vi "lijnvolgen manueel afstandssensor.vi"() -> ()   [LabVIEW 2019]
uses:
  <vilib>/myRIO/Common/Instrument Driver Framework/Utilities/typedefs/Analog Scaling Constants.ctl
  <vilib>/myRIO/Common/Instrument Driver Framework/Utilities/typedefs/Analog Scaling Constants List.ctl
  <vilib>/myRIO/Common/Instrument Driver Framework/myRIO v1.0/AO/typedefs/AO Channels Enum.ctl
  <vilib>/myRIO/Common/Instrument Driver Framework/myRIO v1.0/AO/typedefs/AO Channels List.ctl
  <vilib>/myRIO/Common/Instrument Driver Framework/Utilities/typedefs/Generic FPGA Reference.ctl
  <vilib>/myRIO/Common/Instrument Driver Framework/Utilities/typedefs/myRIO v1.0 Reference.ctl
  <vilib>/myRIO/Common/Instrument Driver Framework/Utilities/typedefs/Hardware Version Enum.ctl
  <vilib>/myRIO/Common/Instrument Driver Framework/Utilities/typedefs/myRIO Generic Hardware Reference.ctl
  <vilib>/myRIO/Instrument Drivers/Onboard IO/AO/typedefs/AO Reference.ctl
  <vilib>/myRIO/Instrument Drivers/Onboard IO/AO/AO.lvlib
  <vilib>/myRIO/Instrument Drivers/Onboard IO/AO/vis/Write.vi
  <vilib>/userDefined/High Color/nirio_resource_hc.ctl
  <vilib>/myRIO/Common/Instrument Driver Framework/myRIO v1.0/AO/vis/myRIO v1.1 Open AO.vi
  <vilib>/myRIO/Instrument Drivers/Onboard IO/AO/vis/myRIO AO Open.xnode
  <vilib>/myRIO/Common/Instrument Driver Framework/Utilities/vis/Is FPGA Ref Available.vi
  <vilib>/myRIO/Express VI/Onboard IO/AO/AO Express VI.xnode
  <vilib>/myRIO/Common/Instrument Driver Framework/myRIO v1.0/AI/typedefs/AI Channels Enum.ctl
  <vilib>/myRIO/Common/Instrument Driver Framework/myRIO v1.0/AI/typedefs/AI Channels List.ctl
  <vilib>/myRIO/Instrument Drivers/Onboard IO/AI/typedefs/AI Reference.ctl
  <vilib>/myRIO/Instrument Drivers/Onboard IO/AI/AI.lvlib
  <vilib>/myRIO/Instrument Drivers/Onboard IO/AI/vis/Read.vi
  <vilib>/myRIO/Common/Instrument Driver Framework/myRIO v1.0/AI/vis/myRIO v1.1 Open AI.vi
  <vilib>/myRIO/Instrument Drivers/Onboard IO/AI/vis/myRIO AI Open.xnode
  <vilib>/myRIO/Express VI/Onboard IO/AI/AI Express VI.xnode
  <vilib>/myRIO/Common/Instrument Driver Framework/myRIO v1.0/DIO/typedefs/DIO Channels Enum.ctl
  <vilib>/myRIO/Common/Instrument Driver Framework/myRIO v1.0/DIO/typedefs/DIO Channels List.ctl
  <vilib>/myRIO/Instrument Drivers/Onboard IO/DIO/typedefs/DIO Reference.ctl
  <vilib>/myRIO/Instrument Drivers/Onboard IO/DIO/DIO.lvlib
  <vilib>/myRIO/Instrument Drivers/Onboard IO/DIO/vis/Read.vi
  <vilib>/myRIO/Common/Instrument Driver Framework/myRIO v1.0/DIO/vis/myRIO v1.1 Open DIO.vi
  <vilib>/myRIO/Instrument Drivers/Onboard IO/DIO/vis/myRIO DIO Open.xnode
  <vilib>/myRIO/Express VI/Onboard IO/DI/DI Express VI.xnode
  Globalmanueel.vi
  <vilib>/myRIO/Instrument Drivers/Onboard IO/DIO/vis/Write.vi
  <vilib>/myRIO/Express VI/Onboard IO/DO/DO Express VI.xnode
panel:
  in  "voorwaarts":bool
  in  "achterwaarts":bool
  in  "links draaien":bool
  in  "rechts draaien":bool
  in  "snelheid":dbl
  in  "links draaien achteruit":bool
  in  "rechts draaien achteruit":bool
  in  "stoppen":bool
  in  "HOOFDWHILELOOP":bool
  out "Numeric 4":i32
  out "analoog":dbl[](array[numeric])
  out "Array 3":i32[](array[numeric])
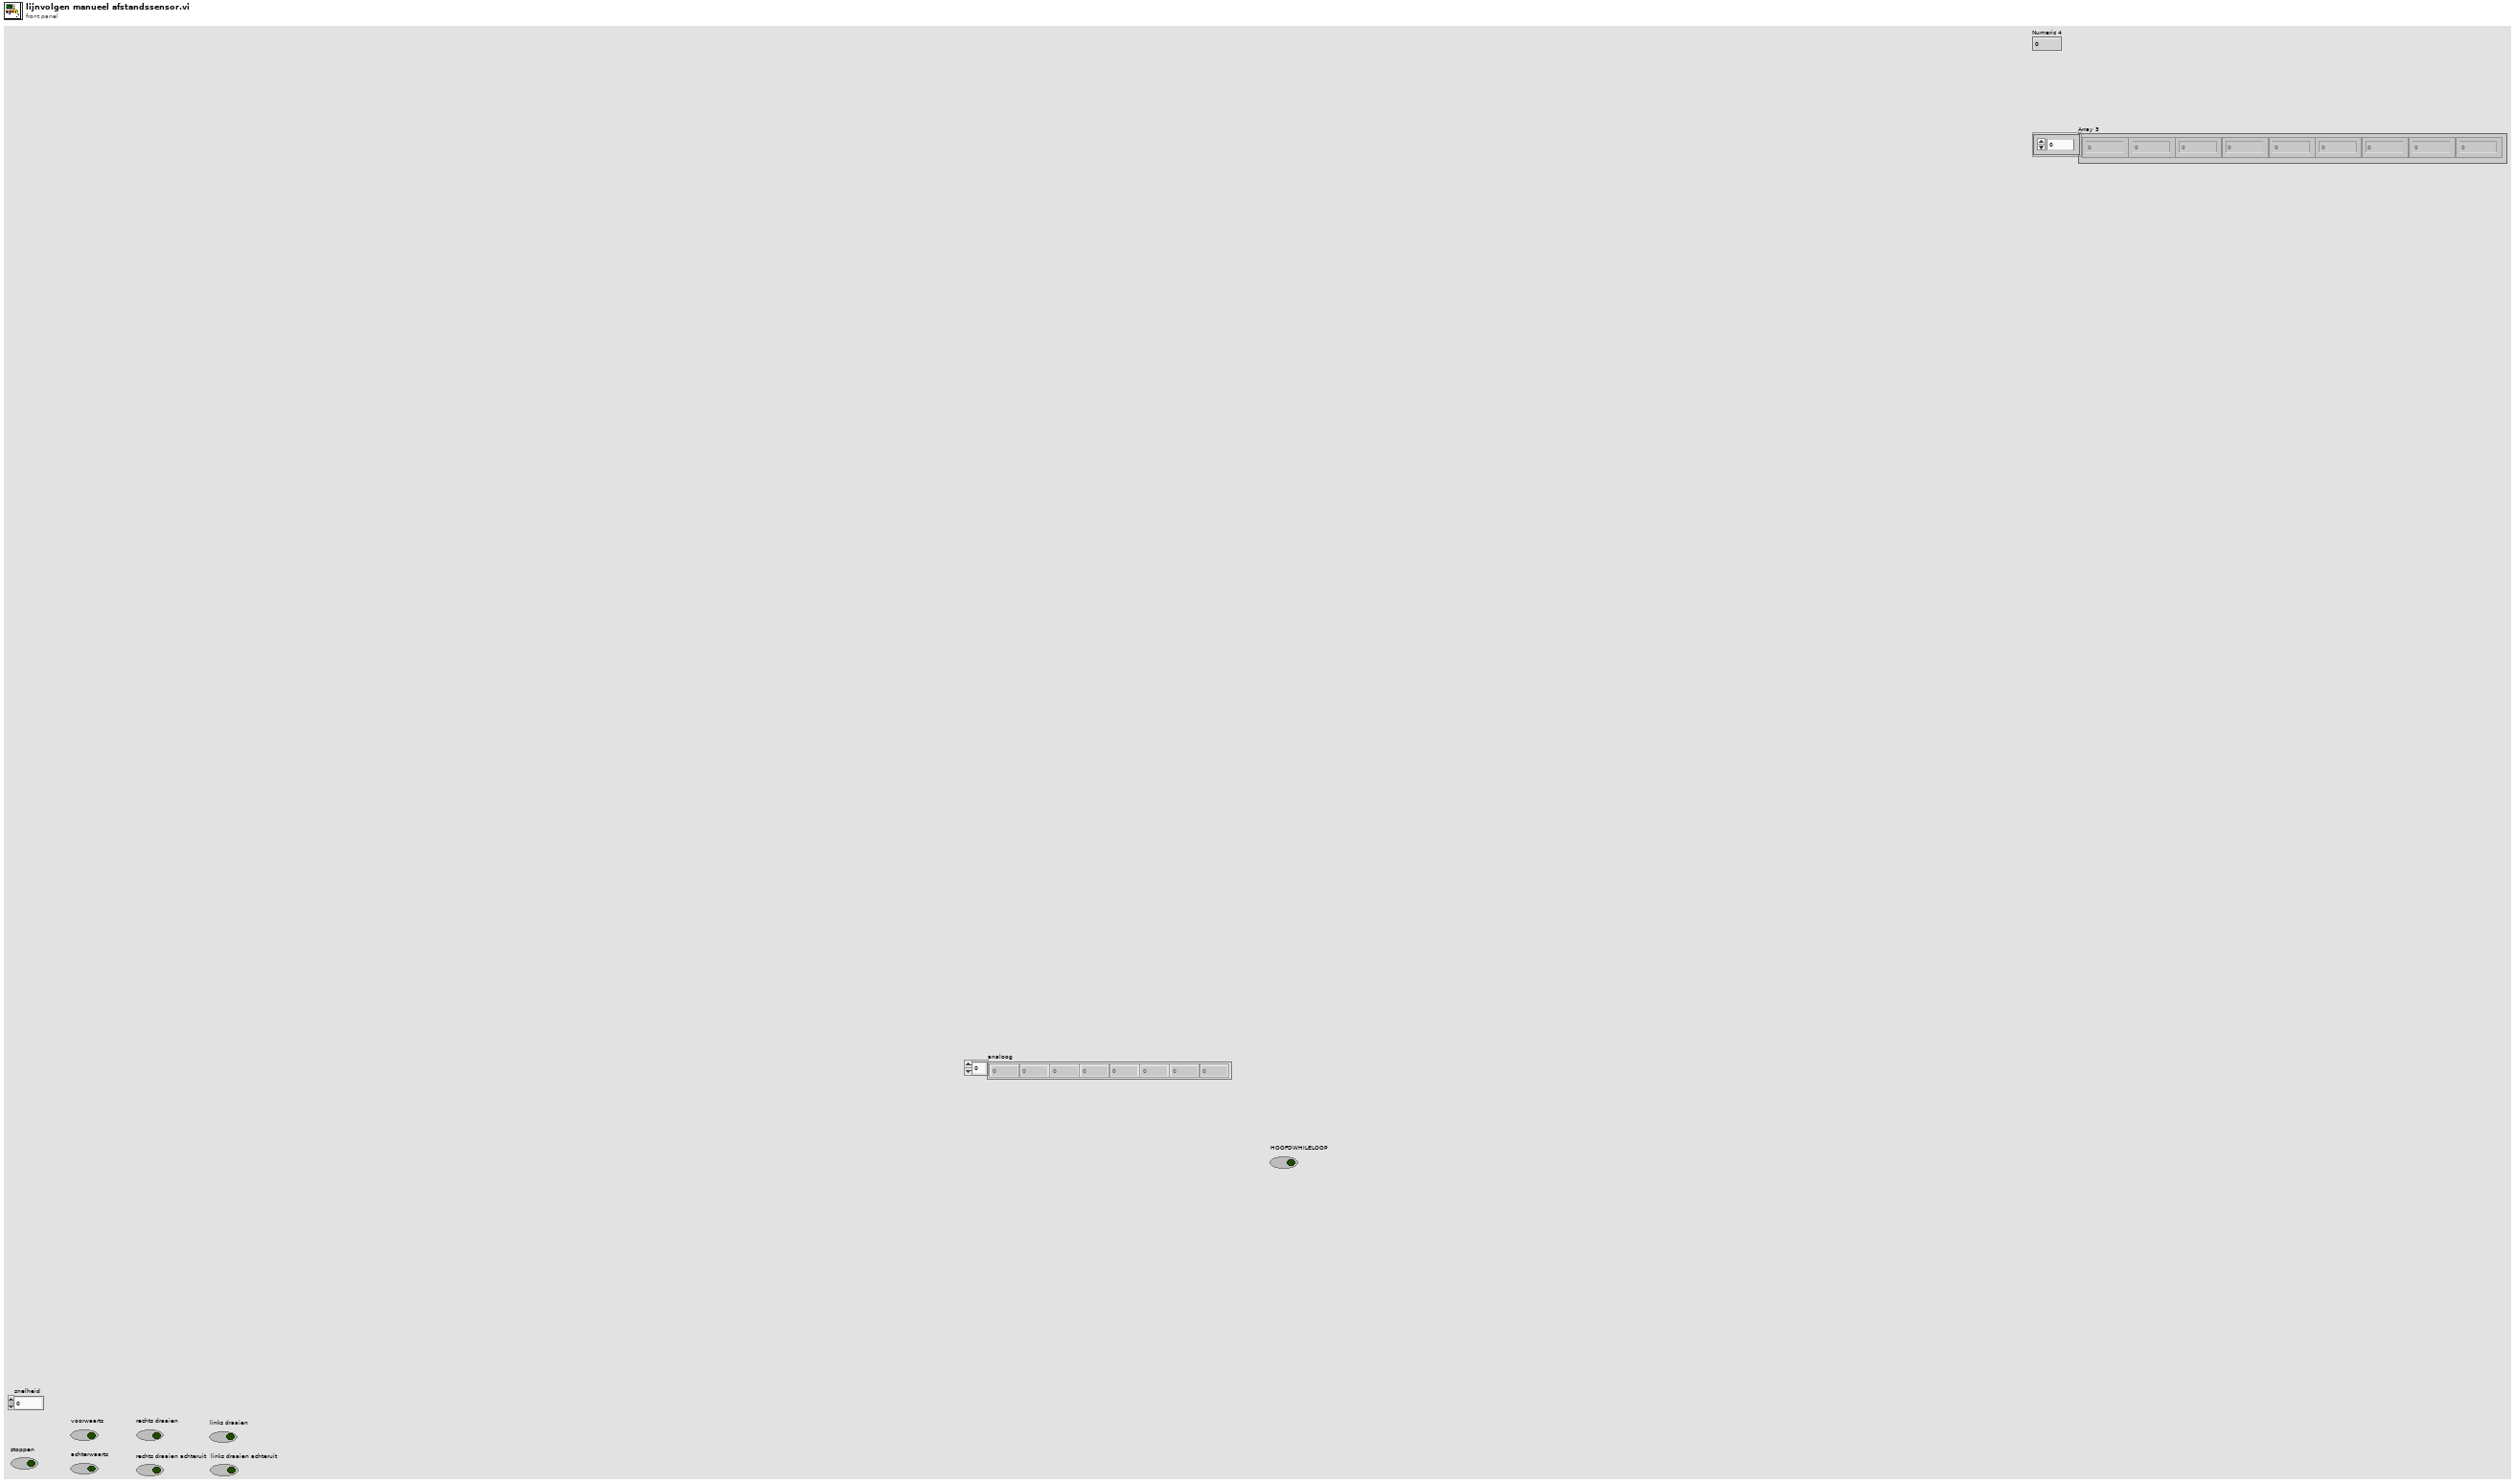
[diagram p1: front panel]
types:
  T1 = typedef "DIO.lvlib/DIO Reference.ctl" = cluster{"myRIO Reference":T2, "DIO Channels List":T6}
  T2 = typedef "myRIO Generic Hardware Reference.ctl" = cluster{"myRIO Model":T3, "myRIO Hardware Reference":T4}
  T3 = typedef "Hardware Version Enum.ctl" = enum16{"Unknown", "myRIO-1900", "myRIO-1950", "roboRIO", "NI ELVIS RIO CM", "ELVIS III"}
  T4 = typedef "myRIO v1.0 Reference.ctl" = cluster{"Generic FPGA Reference":T5, "Allow multiple opens":bool}
  T5 = typedef "Generic FPGA Reference.ctl" = refnum<k20>
  T6 = typedef "DIO Channels List.ctl" = T7[]
  T7 = typedef "DIO Channels Enum.ctl" = enum16{"Not Connected", "C/DIO0", "C/DIO1", "C/DIO2", "C/DIO3", "C/DIO4", "C/DIO5", "C/DIO6", "C/DIO7", "A/DIO0", "A/DIO1", "A/DIO2", "A/DIO3", "A/DIO4", "A/DIO5", "A/DIO6", "A/DIO7", "A/DIO8", "A/DIO9", "A/DIO10", "A/DIO11", "A/DIO12", "A/DIO13", "A/DIO14", "A/DIO15", "A/DIO16", "A/DIO17", "A/DIO18", "A/DIO19", "B/DIO0", "B/DIO1", "B/DIO2", "B/DIO3", "B/DIO4", "B/DIO5", "B/DIO6", "B/DIO7", "B/DIO8", "B/DIO9", "B/DIO10", "B/DIO11", "B/DIO12", "B/DIO13", "B/DIO14", "B/DIO15", "B/DIO16", "B/DIO17", "B/DIO18", "B/DIO19", "LED0", "LED1", "LED2", "LED3", "Button0", "DIO/DIO0", "DIO/DIO1", "DIO/DIO2", "DIO/DIO3", "DIO/DIO4", "DIO/DIO5", "DIO/DIO6", "DIO/DIO7", "DIO/DIO8", "DIO/DIO9", "SPI/CS0", "SPI/CS1", "SPI/CS2", "SPI/CS3", "LED RADIO (Green)", "LED RADIO (Red)", "LED COMM (Green)", "LED COMM (Red)", "LED MODE (Green)", "LED MODE (Red)"}
  T8 = typedef "nirio_resource_hc.ctl" = tag
  T9 = typedef "AO.lvlib/AO Reference.ctl" = cluster{"myRIO Reference":T2, "AO Channel List":T10, "AO Scaling Constant List":T12}
  T10 = typedef "AO Channels List.ctl" = T11[]
  T11 = typedef "AO Channels Enum.ctl" = enum16{"Not Connected", "AudioOut/Left", "AudioOut/Right", "C/AO0", "C/AO1", "A/AO0", "A/AO1", "B/AO0", "B/AO1"}
  T12 = typedef "Analog Scaling Constants List.ctl" = T13[]
  T13 = typedef "Analog Scaling Constants.ctl" = cluster{"LSB Weight (Volts)":dbl, "Offset (Volts)":dbl, "Signed?":bool}
  T14 = typedef "AI.lvlib/AI Reference.ctl" = cluster{"myRIO Reference":T2, "AI Channels List":T15, "AI Scaling Constants List":T12}
  T15 = typedef "AI Channels List.ctl" = T16[]
  T16 = typedef "AI Channels Enum.ctl" = enum16{"Not Connected", "AudioIn/Left", "AudioIn/Right", "C/AI0", "C/AI1", "A/AI0", "A/AI1", "A/AI2", "A/AI3", "A/AI4", "A/AI5", "A/AI6", "A/AI7", "B/AI0", "B/AI1", "B/AI2", "B/AI3", "B/AI4", "B/AI5", "B/AI6", "B/AI7", "AI/AI0", "AI/AI1", "AI/AI2", "AI/AI3", "A/AI0 (DIFF)", "A/AI1 (DIFF)", "A/AI2 (DIFF)", "A/AI3 (DIFF)", "B/AI0 (DIFF)", "B/AI1 (DIFF)", "B/AI2 (DIFF)", "B/AI3 (DIFF)"}
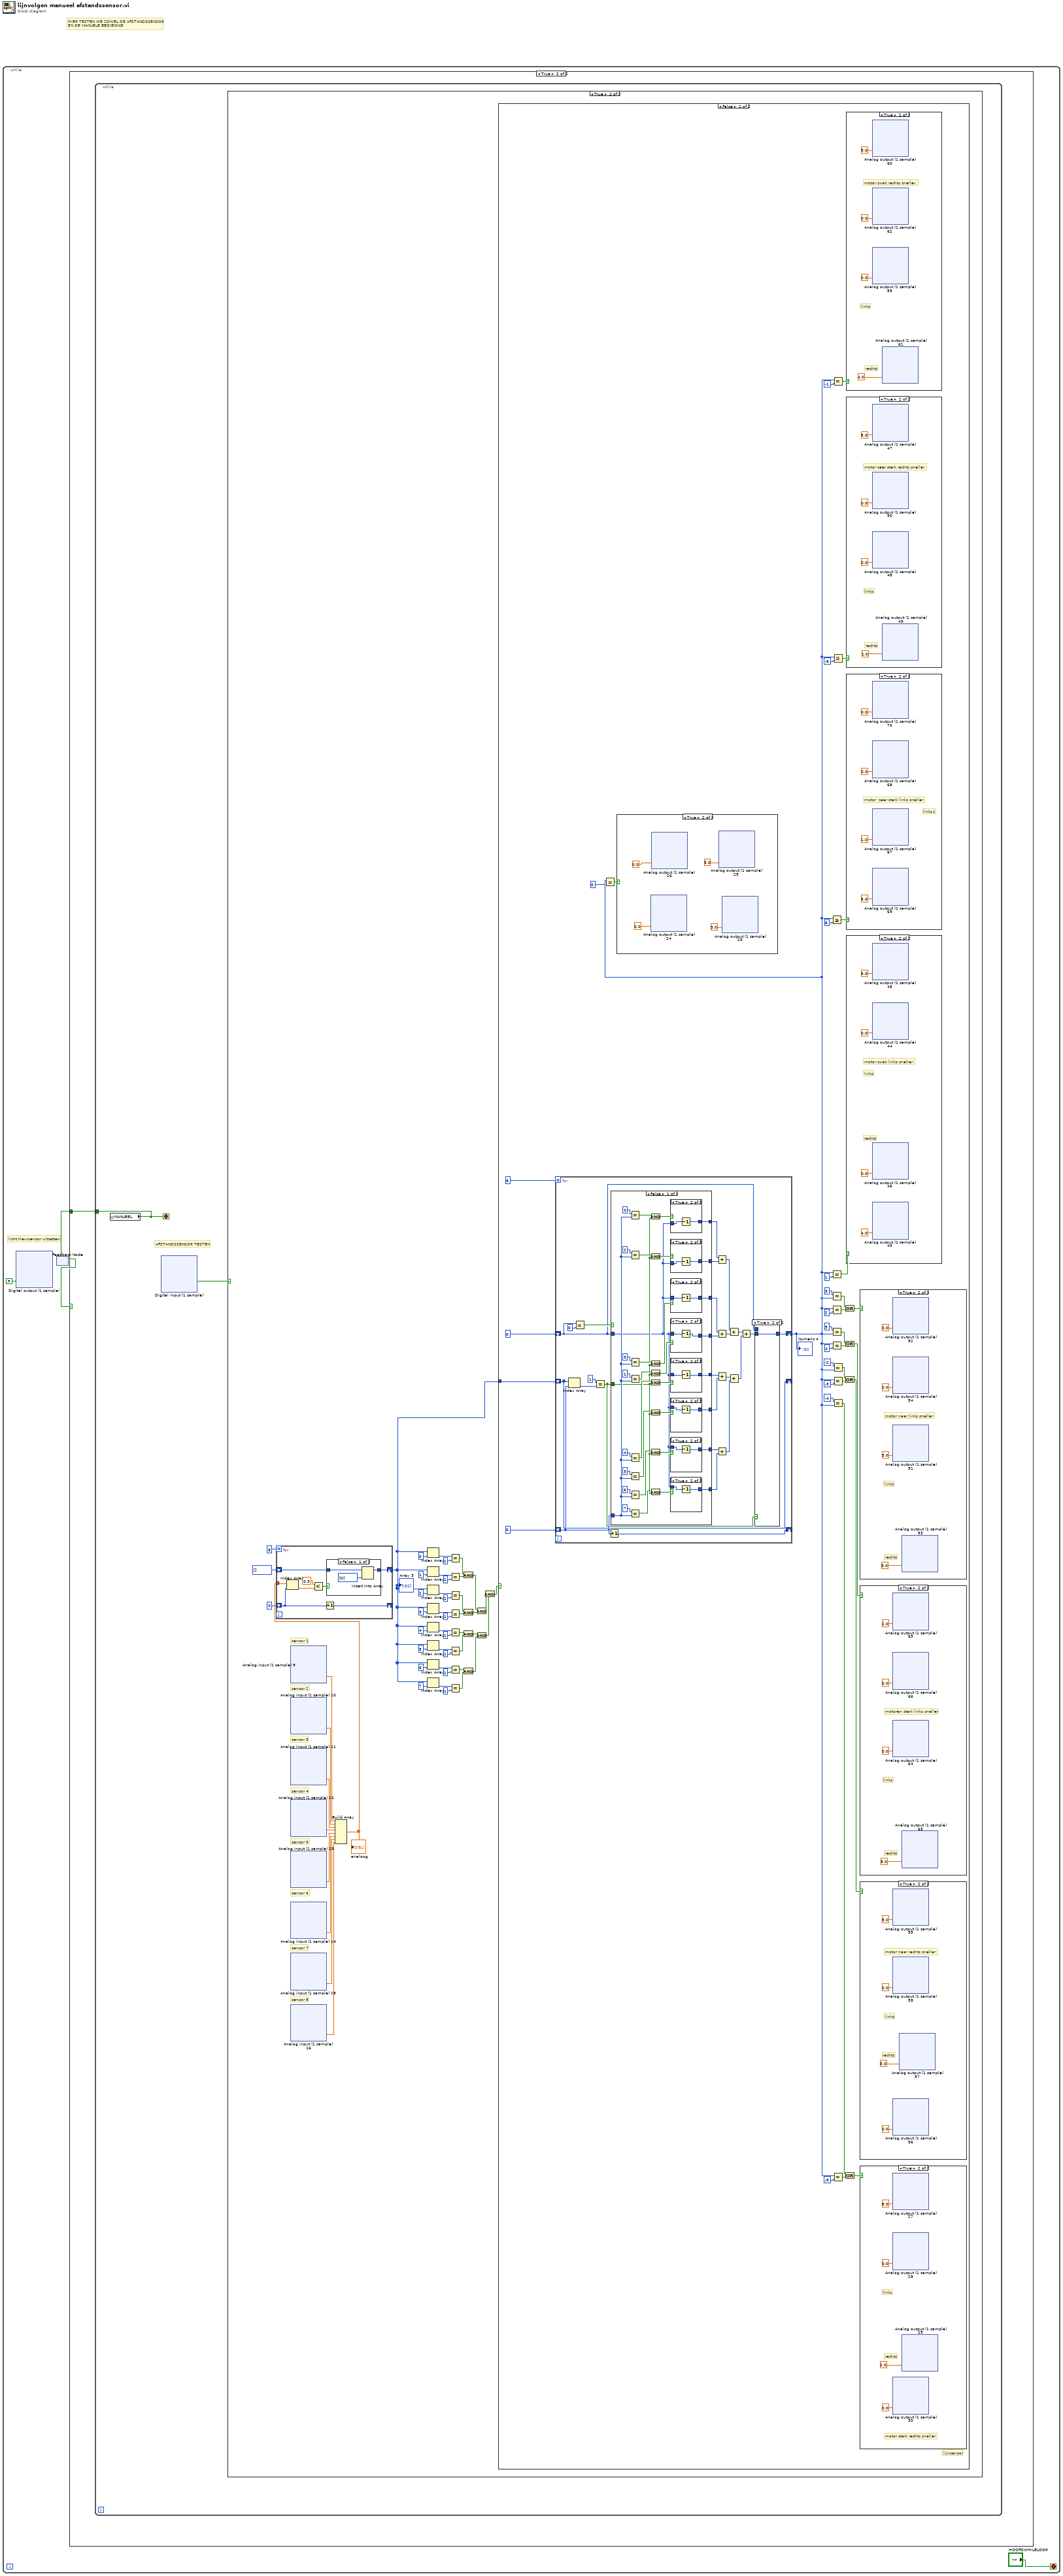
[diagram p0: block diagram]
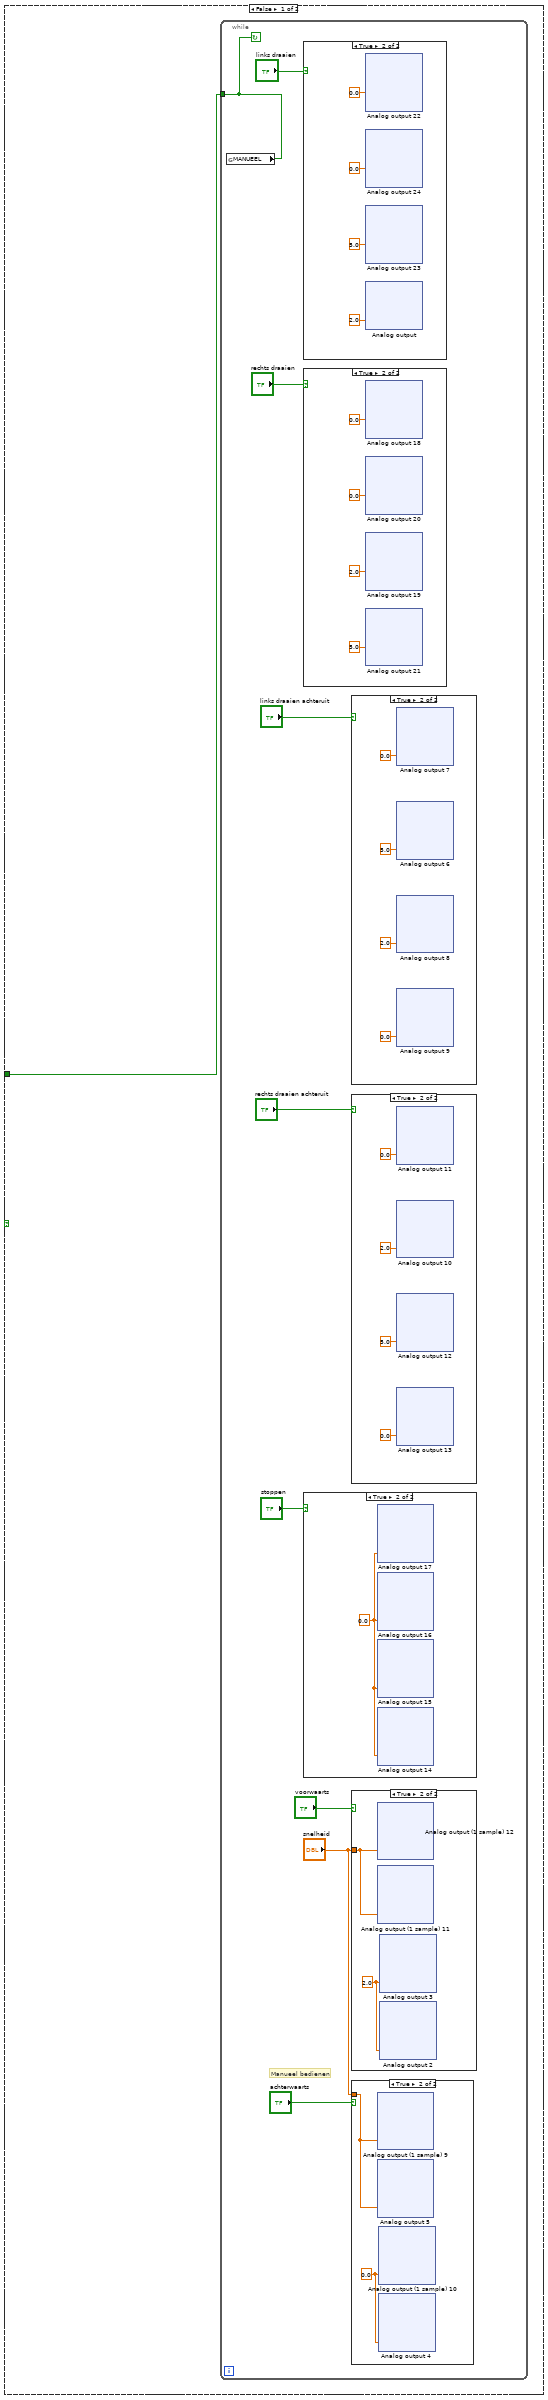
[diagram p2: hidden frame]
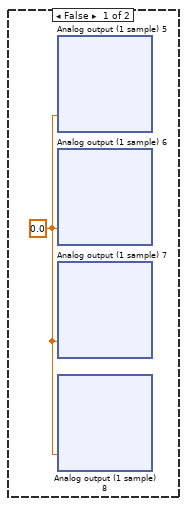
[diagram p10: hidden frame]
diagram:
  # "HIER TESTEN WE ZOWEL DE AFSTANDSSENSOR\nEN DE MANUELE BEDIENING"
  n1 = while {
    stop <- "HOOFDWHILELOOP" stop-if-true
    # "licht kleursensor uitzetten"
    n2 = xnode "Digital output (1 sample)"("A/DIO2 (Pin 15)"=FALSE) -> ()  [unwired: 1 in, 1 out]
    n3 = feedback #1() -> (w1:bool)  [unwired: 1 in]
    n4 = case shown="True" w1 {
      tunnel: [w40 w1107] -> w2
      frame False {
        n5 = while {
          tunnel: [w41] -> w40
          stop <- w41 continue-if-true
          # "Manueel bedienen"
          n6 = global read "Globalmanueel.vi" "MANUEEL"() -> (w41:bool)
          n7 = case shown="True" "links draaien" {
            frame False {
            }
            frame True {
              n8 = xnode "Analog output 22"("B/AO1 (Pin 4)"=0.0) -> ()  [unwired: 1 in, 1 out]
              n9 = xnode "Analog output 24"("A/AO1 (Pin 4)"=0.0) -> ()  [unwired: 1 in, 1 out]
              n10 = xnode "Analog output 23"("B/AO0 (Pin 2)"=5.0) -> ()  [unwired: 1 in, 1 out]
              n11 = xnode "Analog output"("A/AO0 (Pin 2)"=2.0) -> ()  [unwired: 1 in, 1 out]
            }
          }
          n12 = case shown="True" "rechts draaien" {
            frame False {
            }
            frame True {
              n13 = xnode "Analog output 18"("B/AO1 (Pin 4)"=0.0) -> ()  [unwired: 1 in, 1 out]
              n14 = xnode "Analog output 20"("A/AO1 (Pin 4)"=0.0) -> ()  [unwired: 1 in, 1 out]
              n15 = xnode "Analog output 19"("B/AO0 (Pin 2)"=2.0) -> ()  [unwired: 1 in, 1 out]
              n16 = xnode "Analog output 21"("A/AO0 (Pin 2)"=5.0) -> ()  [unwired: 1 in, 1 out]
            }
          }
          n17 = case shown="True" "stoppen" {
            frame False {
            }
            frame True {
              w50 = 0.0
              n18 = xnode "Analog output 17"("A/AO0 (Pin 2)"=w50) -> ()  [unwired: 1 in, 1 out]
              n19 = xnode "Analog output 16"("A/AO1 (Pin 4)"=w50) -> ()  [unwired: 1 in, 1 out]
              n20 = xnode "Analog output 15"("B/AO0 (Pin 2)"=w50) -> ()  [unwired: 1 in, 1 out]
              n21 = xnode "Analog output 14"("B/AO1 (Pin 4)"=w50) -> ()  [unwired: 1 in, 1 out]
            }
          }
          n22 = case shown="True" "links draaien achteruit" {
            frame False {
            }
            frame True {
              n23 = xnode "Analog output 7"("B/AO0 (Pin 2)"=0.0) -> ()  [unwired: 1 in, 1 out]
              n24 = xnode "Analog output 6"("B/AO1 (Pin 4)"=5.0) -> ()  [unwired: 1 in, 1 out]
              n25 = xnode "Analog output 8"("A/AO1 (Pin 4)"=2.0) -> ()  [unwired: 1 in, 1 out]
              n26 = xnode "Analog output 9"("A/AO0 (Pin 2)"=0.0) -> ()  [unwired: 1 in, 1 out]
            }
          }
          n27 = case shown="True" "rechts draaien achteruit" {
            frame False {
            }
            frame True {
              n28 = xnode "Analog output 11"("B/AO0 (Pin 2)"=0.0) -> ()  [unwired: 1 in, 1 out]
              n29 = xnode "Analog output 10"("B/AO1 (Pin 4)"=2.0) -> ()  [unwired: 1 in, 1 out]
              n30 = xnode "Analog output 12"("A/AO1 (Pin 4)"=5.0) -> ()  [unwired: 1 in, 1 out]
              n31 = xnode "Analog output 13"("A/AO0 (Pin 2)"=0.0) -> ()  [unwired: 1 in, 1 out]
            }
          }
          n32 = case shown="True" "voorwaarts" {
            tunnel: "snelheid" -> [_ w957]
            frame False {
            }
            frame True {
              w958 = 2.0
              n33 = xnode "Analog output (1 sample) 12"("A/AO0 (Pin 2)"=w957) -> ()  [unwired: 1 in, 1 out]
              n34 = xnode "Analog output (1 sample) 11"("B/AO0 (Pin 2)"=w957) -> ()  [unwired: 1 in, 1 out]
              n35 = xnode "Analog output 3"("A/AO1 (Pin 4)"=w958) -> ()  [unwired: 1 in, 1 out]
              n36 = xnode "Analog output 2"("B/AO1 (Pin 4)"=w958) -> ()  [unwired: 1 in, 1 out]
            }
          }
          n37 = case shown="True" "achterwaarts" {
            tunnel: "snelheid" -> [_ w807]
            frame False {
            }
            frame True {
              w808 = 0.0
              n38 = xnode "Analog output (1 sample) 9"("A/AO1 (Pin 4)"=w807) -> ()  [unwired: 1 in, 1 out]
              n39 = xnode "Analog output 5"("B/AO1 (Pin 4)"=w807) -> ()  [unwired: 1 in, 1 out]
              n40 = xnode "Analog output (1 sample) 10"("A/AO0 (Pin 2)"=w808) -> ()  [unwired: 1 in, 1 out]
              n41 = xnode "Analog output 4"("B/AO0 (Pin 2)"=w808) -> ()  [unwired: 1 in, 1 out]
            }
          }
        }
      }
      frame True {
        n42 = while {
          tunnel: [w1108] -> w1107
          stop <- w1108 stop-if-true
          # "AFSTANDSSENSOR TESTEN"
          n43 = global read "Globalmanueel.vi" "MANUEEL"() -> (w1108:bool)
          n44 = xnode "Digital input (1 sample)"() -> ("A/DIO1 (Pin 13)"=w1109:bool)  [unwired: 1 in, 1 out]
          n45 = case shown="True" w1109 {
            frame False {
              w1145 = 0.0
              n46 = xnode "Analog output (1 sample) 5"("A/AO0 (Pin 2)"=w1145) -> ()  [unwired: 1 in, 1 out]
              n47 = xnode "Analog output (1 sample) 6"("A/AO1 (Pin 4)"=w1145) -> ()  [unwired: 1 in, 1 out]
              n48 = xnode "Analog output (1 sample) 7"("B/AO0 (Pin 2)"=w1145) -> ()  [unwired: 1 in, 1 out]
              n49 = xnode "Analog output (1 sample) 8"("B/AO1 (Pin 4)"=w1145) -> ()  [unwired: 1 in, 1 out]
            }
            frame True {
              # "sensor 8"
              # "sensor 7"
              # "sensor 6"
              # "sensor 5"
              # "sensor 4"
              # "sensor 3"
              # "sensor 2"
              # "sensor 1"
              n50 = xnode "Analog input (1 sample) 9"() -> ("A/AI3 (Pin 9)"=w1297:dbl)  [unwired: 1 in, 1 out]
              n51 = xnode "Analog input (1 sample) 10"() -> ("A/AI2 (Pin 7)"=w1298:dbl)  [unwired: 1 in, 1 out]
              n52 = xnode "Analog input (1 sample) 11"() -> ("A/AI1 (Pin 5)"=w1299:dbl)  [unwired: 1 in, 1 out]
              n53 = xnode "Analog input (1 sample) 12"() -> ("A/AI0 (Pin 3)"=w1300:dbl)  [unwired: 1 in, 1 out]
              n54 = xnode "Analog input (1 sample) 13"() -> ("B/AI3 (Pin 9)"=w1301:dbl)  [unwired: 1 in, 1 out]
              n55 = xnode "Analog input (1 sample) 14"() -> ("B/AI2 (Pin 7)"=w1302:dbl)  [unwired: 1 in, 1 out]
              n56 = xnode "Analog input (1 sample) 15"() -> ("A/AI1 (Pin 5)"=w1303:dbl)  [unwired: 1 in, 1 out]
              n57 = xnode "Analog input (1 sample) 16"() -> ("B/AI0 (Pin 3)"=w1304:dbl)  [unwired: 1 in, 1 out]
              n58 = Build Array(w1297, w1298, w1299, w1300, w1301, w1302, w1303, w1304) -> (w1296:dbl[])
              "analoog" <- w1296
              n59 = for {
                N: 8 -> [_]
                shift-right: [w3386] -> w1294
                shift-left: i32[] [] -> [w3387]
                shift-right: [w3383] -> _
                shift-left: 0 -> [w3382]
                tunnel: w1296 -> [w3380]
                n60 = Index Array(array=w3380, index=w3382) -> (element=w3381:dbl)
                n61 = Less?(x=0.3, y=w3381) -> (x < y?=w3385:bool)
                n62 = Increment(x=w3382) -> (x+1=w3383:i32)
                n63 = case shown="False" w3385 {
                  tunnel: w3387 -> [w3389 w3391]
                  tunnel: [w3390 w3393] -> w3386
                  frame False {
                    n64 = Insert Into Array(array=w3389, new element=i32[] [0]) -> (w3390:i32[])  [unwired: 1 in]
                  }
                  frame True {
                    n65 = Insert Into Array(array=w3391, new element=i32[] [1, 1]) -> (w3393:i32[])  [unwired: 1 in]
                  }
                }
              }
              "Array 3" <- w1294
              n66 = Index Array(array=w1294, index=0) -> (element=w1326:i32)
              n67 = Index Array(array=w1294, index=1) -> (element=w1305:i32)
              n68 = Index Array(array=w1294, index=2) -> (element=w1311:i32)
              n69 = Index Array(array=w1294, index=3) -> (element=w1308:i32)
              n70 = Index Array(array=w1294, index=4) -> (element=w1314:i32)
              n71 = Index Array(array=w1294, index=5) -> (element=w1317:i32)
              n72 = Index Array(array=w1294, index=6) -> (element=w1320:i32)
              n73 = Index Array(array=w1294, index=7) -> (element=w1323:i32)
              n74 = Equal?(x=w1326, y=1) -> (x = y?=w1329:bool)
              n75 = Equal?(x=w1305, y=1) -> (x = y?=w1330:bool)
              n76 = Equal?(x=w1311, y=1) -> (x = y?=w1331:bool)
              n77 = Equal?(x=w1308, y=1) -> (x = y?=w1332:bool)
              n78 = Equal?(x=w1314, y=1) -> (x = y?=w1333:bool)
              n79 = Equal?(x=w1317, y=1) -> (x = y?=w1334:bool)
              n80 = Equal?(x=w1320, y=1) -> (x = y?=w1335:bool)
              n81 = Equal?(x=w1323, y=1) -> (x = y?=w1336:bool)
              n82 = And(x=w1329, y=w1330) -> (x .and. y?=w1337:bool)
              n83 = And(x=w1331, y=w1332) -> (x .and. y?=w1338:bool)
              n84 = And(x=w1333, y=w1334) -> (x .and. y?=w1339:bool)
              n85 = And(x=w1335, y=w1336) -> (x .and. y?=w1340:bool)
              n86 = And(x=w1337, y=w1338) -> (x .and. y?=w1341:bool)
              n87 = And(x=w1339, y=w1340) -> (x .and. y?=w1342:bool)
              n88 = And(x=w1341, y=w1342) -> (x .and. y?=w1295:bool)
              n89 = case shown="False" w1295 {
                tunnel: w1294 -> [w1346 _]
                frame False {
                  # "lijnsensor"
                  n90 = for {
                    N: 8 -> [_]
                    shift-right: [w2759] -> _
                    shift-left: 0 -> [w2773]
                    shift-right: [w2751] -> w1347
                    shift-left: 0 -> [w2752]
                    shift-right: [w2764] -> _
                    shift-left: w1346 -> [w2764]
                    n91 = Index Array(array=w2764, index=w2773) -> (element=w2763:i32)
                    n92 = Equal?(x=w2752, y=0) -> (x = y?=w2760:bool)
                    n93 = Equal?(x=1, y=w2763) -> (x = y?=w2750:bool)
                    n94 = Increment(x=w2773) -> (x+1=w2759:i32)
                    n95 = case shown="False" w2760 {
                      tunnel: w2773 -> [w2783 w2869]
                      tunnel: [w2777 w2868] -> w2772
                      tunnel: [w2784 w2867] -> w2771
                      tunnel: [w2785 w2866] -> w2770
                      tunnel: [w2786 w2865] -> w2769
                      tunnel: w2752 -> [w2776 w2864]
                      tunnel: w2750 -> [w2782 w2855]
                      tunnel: [w2780 w2854] -> w2758
                      tunnel: [w2781 w2853] -> w2757
                      tunnel: [w2778 w2852] -> w2755
                      tunnel: [w2779 w2851] -> w2754
                      frame False {
                        n96 = Equal?(x=0, y=w2783) -> (x = y?=w2803:bool)
                        n97 = Equal?(x=2, y=w2783) -> (x = y?=w2809:bool)
                        n98 = Equal?(x=3, y=w2783) -> (x = y?=w2810:bool)
                        n99 = Equal?(x=1, y=w2783) -> (x = y?=w2795:bool)
                        n100 = Equal?(x=4, y=w2783) -> (x = y?=w2807:bool)
                        n101 = Equal?(x=5, y=w2783) -> (x = y?=w2808:bool)
                        n102 = Equal?(x=6, y=w2783) -> (x = y?=w2806:bool)
                        n103 = Equal?(x=7, y=w2783) -> (x = y?=w2805:bool)
                        n104 = And(x=w2803, y=w2782) -> (x .and. y?=w2787:bool)
                        n105 = And(x=w2809, y=w2782) -> (x .and. y?=w2789:bool)
                        n106 = And(x=w2810, y=w2782) -> (x .and. y?=w2790:bool)
                        n107 = And(x=w2795, y=w2782) -> (x .and. y?=w2788:bool)
                        n108 = And(x=w2807, y=w2782) -> (x .and. y?=w2791:bool)
                        n109 = And(x=w2808, y=w2782) -> (x .and. y?=w2792:bool)
                        n110 = And(x=w2806, y=w2782) -> (x .and. y?=w2793:bool)
                        n111 = And(x=w2805, y=w2782) -> (x .and. y?=w2794:bool)
                        n112 = case shown="True" w2787 {
                          tunnel: [w2812 w2815] -> w2781
                          tunnel: w2776 -> [w2811 w2814]
                          frame False {
                            n113 = Multiply(x=0, y=w2811) -> (x*y=w2812:i32)
                          }
                          frame True {
                            n114 = Decrement(x=w2814) -> (x-1=w2815:i32)
                          }
                        }
                        n115 = case shown="True" w2789 {
                          tunnel: [w2843 w2844] -> w2780
                          tunnel: w2776 -> [w2842 w2845]
                          frame False {
                            n116 = Multiply(x=0, y=w2842) -> (x*y=w2843:i32)
                          }
                          frame True {
                            n117 = Decrement(x=w2845) -> (x-1=w2844:i32)
                          }
                        }
                        n118 = case shown="True" w2790 {
                          tunnel: [w2837 w2840] -> w2779
                          tunnel: w2776 -> [w2836 w2839]
                          frame False {
                            n119 = Multiply(x=0, y=w2836) -> (x*y=w2837:i32)
                          }
                          frame True {
                            n120 = Decrement(x=w2839) -> (x-1=w2840:i32)
                          }
                        }
                        n121 = case shown="True" w2788 {
                          tunnel: [w2847 w2850] -> w2778
                          tunnel: w2776 -> [w2846 w2849]
                          frame False {
                            n122 = Multiply(x=0, y=w2846) -> (x*y=w2847:i32)
                          }
                          frame True {
                            n123 = Decrement(x=w2849) -> (x-1=w2850:i32)
                          }
                        }
                        n124 = case shown="True" w2791 {
                          tunnel: [w2832 w2835] -> w2777
                          tunnel: w2776 -> [w2831 w2834]
                          frame False {
                            n125 = Multiply(x=0, y=w2831) -> (x*y=w2832:i32)
                          }
                          frame True {
                            n126 = Decrement(x=w2834) -> (x-1=w2835:i32)
                          }
                        }
                        n127 = case shown="True" w2792 {
                          tunnel: [w2822 w2825] -> w2784
                          tunnel: w2776 -> [w2821 w2824]
                          frame False {
                            n128 = Multiply(x=0, y=w2821) -> (x*y=w2822:i32)
                          }
                          frame True {
                            n129 = Decrement(x=w2824) -> (x-1=w2825:i32)
                          }
                        }
                        n130 = case shown="True" w2793 {
                          tunnel: [w2827 w2830] -> w2785
                          tunnel: w2776 -> [w2826 w2829]
                          frame False {
                            n131 = Multiply(x=0, y=w2826) -> (x*y=w2827:i32)
                          }
                          frame True {
                            n132 = Decrement(x=w2829) -> (x-1=w2830:i32)
                          }
                        }
                        n133 = case shown="True" w2794 {
                          tunnel: [w2816 w2820] -> w2786
                          tunnel: w2776 -> [w2817 w2819]
                          frame False {
                            n134 = Multiply(x=0, y=w2817) -> (x*y=w2816:i32)
                          }
                          frame True {
                            n135 = Decrement(x=w2819) -> (x-1=w2820:i32)
                          }
                        }
                      }
                      frame True {
                        n136 = Equal?(x=0, y=w2869) -> (x = y?=w2878:bool)
                        n137 = Equal?(x=1, y=w2869) -> (x = y?=w2870:bool)
                        n138 = Equal?(x=2, y=w2869) -> (x = y?=w2884:bool)
                        n139 = Equal?(x=3, y=w2869) -> (x = y?=w2885:bool)
                        n140 = Equal?(x=4, y=w2869) -> (x = y?=w2882:bool)
                        n141 = Equal?(x=5, y=w2869) -> (x = y?=w2883:bool)
                        n142 = Equal?(x=6, y=w2869) -> (x = y?=w2881:bool)
                        n143 = Equal?(x=7, y=w2869) -> (x = y?=w2880:bool)
                        n144 = And(x=w2878, y=w2855) -> (x .and. y?=w2856:bool)
                        n145 = And(x=w2870, y=w2855) -> (x .and. y?=w2857:bool)
                        n146 = And(x=w2884, y=w2855) -> (x .and. y?=w2858:bool)
                        n147 = And(x=w2885, y=w2855) -> (x .and. y?=w2859:bool)
                        n148 = And(x=w2882, y=w2855) -> (x .and. y?=w2860:bool)
                        n149 = And(x=w2883, y=w2855) -> (x .and. y?=w2861:bool)
                        n150 = And(x=w2881, y=w2855) -> (x .and. y?=w2862:bool)
                        n151 = And(x=w2880, y=w2855) -> (x .and. y?=w2863:bool)
                        n152 = case shown="True" w2856 {
                          tunnel: w2864 -> [w2886 w2890]
                          tunnel: [w2887 w2889] -> w2853
                          frame False {
                            n153 = Multiply(x=0, y=w2886) -> (x*y=w2887:i32)
                          }
                          frame True {
                            n154 = Add(x=7, y=w2890) -> (x+y=w2889:i32)
                          }
                        }
                        n155 = case shown="True" w2857 {
                          tunnel: w2864 -> [w2926 w2929]
                          tunnel: [w2927 w2930] -> w2854
                          frame False {
                            n156 = Multiply(x=0, y=w2926) -> (x*y=w2927:i32)
                          }
                          frame True {
                            n157 = Add(x=5, y=w2929) -> (x+y=w2930:i32)
                          }
                        }
                        n158 = case shown="True" w2858 {
                          tunnel: w2864 -> [w2920 w2924]
                          tunnel: [w2921 w2923] -> w2851
                          frame False {
                            n159 = Multiply(x=0, y=w2920) -> (x*y=w2921:i32)
                          }
                          frame True {
                            n160 = Add(x=3, y=w2924) -> (x+y=w2923:i32)
                          }
                        }
                        n161 = case shown="True" w2859 {
                          tunnel: w2864 -> [w2916 w2919]
                          tunnel: [w2915 w2918] -> w2852
                          frame False {
                            n162 = Multiply(x=0, y=w2916) -> (x*y=w2915:i32)
                          }
                          frame True {
                            n163 = Increment(x=w2919) -> (x+1=w2918:i32)
                          }
                        }
                        n164 = case shown="True" w2860 {
                          tunnel: w2864 -> [w2910 w2914]
                          tunnel: [w2911 w2913] -> w2868
                          frame False {
                            n165 = Multiply(x=0, y=w2910) -> (x*y=w2911:i32)
                          }
                          frame True {
                            n166 = Decrement(x=w2914) -> (x-1=w2913:i32)
                          }
                        }
                        n167 = case shown="True" w2861 {
                          tunnel: w2864 -> [w2899 w2901]
                          tunnel: [w2898 w2903] -> w2867
                          frame False {
                            n168 = Multiply(x=0, y=w2899) -> (x*y=w2898:i32)
                          }
                          frame True {
                            n169 = Subtract(x=w2901, y=3) -> (x-y=w2903:i32)
                          }
                        }
                        n170 = case shown="True" w2862 {
                          tunnel: w2864 -> [w2905 w2907]
                          tunnel: [w2904 w2908] -> w2866
                          frame False {
                            n171 = Multiply(x=0, y=w2905) -> (x*y=w2904:i32)
                          }
                          frame True {
                            n172 = Subtract(x=w2907, y=5) -> (x-y=w2908:i32)
                          }
                        }
                        n173 = case shown="True" w2863 {
                          tunnel: w2864 -> [w2892 w2895]
                          tunnel: [w2893 w2896] -> w2865
                          frame False {
                            n174 = Multiply(x=0, y=w2892) -> (x*y=w2893:i32)
                          }
                          frame True {
                            n175 = Subtract(x=w2895, y=7) -> (x-y=w2896:i32)
                          }
                        }
                      }
                    }
                    n176 = Add(x=w2757, y=w2758) -> (x+y=w2756:i32)
                    n177 = Add(x=w2754, y=w2755) -> (x+y=w2753:i32)
                    n178 = Add(x=w2772, y=w2771) -> (x+y=w2767:i32)
                    n179 = Add(x=w2770, y=w2769) -> (x+y=w2768:i32)
                    n180 = Add(x=w2756, y=w2753) -> (x+y=w2766:i32)
                    n181 = Add(x=w2767, y=w2768) -> (x+y=w2765:i32)
                    n182 = Add(x=w2766, y=w2765) -> (x+y=w2749:i32)
                    n183 = case shown="True" w2750 {
                      tunnel: w2752 -> [w2774 _]
                      tunnel: [w2774 w2775] -> w2751
                      tunnel: w2749 -> [_ w2775]
                      frame False {
                      }
                      frame True {
                      }
                    }
                  }
                  "Numeric 4" <- w1347
                  n184 = Equal?(x=w1347, y=0) -> (x = y?=w1349:bool)
                  n185 = case shown="True" w1349 {
                    frame False {
                    }
                    frame True {
                      n186 = xnode "Analog output (1 sample) 24"("B/AO0 (Pin 2)"=0.0) -> ()  [unwired: 1 in, 1 out]
                      n187 = xnode "Analog output (1 sample) 26"("A/AO0 (Pin 2)"=0.0) -> ()  [unwired: 1 in, 1 out]
                      n188 = xnode "Analog output (1 sample) 25"("A/AO1 (Pin 4)"=3.0) -> ()  [unwired: 1 in, 1 out]
                      n189 = xnode "Analog output (1 sample) 23"("B/AO1 (Pin 4)"=3.0) -> ()  [unwired: 1 in, 1 out]
                    }
                  }
                  n190 = Greater Or Equal?(x=w1347, y=6) -> (x >= y?=w1375:bool)
                  n191 = Equal?(x=w1347, y=1) -> (x = y?=w1376:bool)
                  n192 = Equal?(x=3, y=w1347) -> (x = y?=w1366:bool)
                  n193 = Equal?(x=w1347, y=2) -> (x = y?=w1367:bool)
                  n194 = Equal?(x=5, y=w1347) -> (x = y?=w1370:bool)
                  n195 = Equal?(x=w1347, y=4) -> (x = y?=w1371:bool)
                  n196 = Equal?(x=w1347, y=-1) -> (x = y?=w1354:bool)
                  n197 = Less Or Equal?(x=w1347, y=-6) -> (x <= y?=w1352:bool)
                  n198 = Equal?(x=-2, y=w1347) -> (x = y?=w1360:bool)
                  n199 = Equal?(x=w1347, y=-3) -> (x = y?=w1361:bool)
                  n200 = Equal?(x=-4, y=w1347) -> (x = y?=w1356:bool)
                  n201 = Equal?(x=w1347, y=-5) -> (x = y?=w1357:bool)
                  n202 = Or(x=w1366, y=w1367) -> (x .or. y?=w1364:bool)
                  n203 = Or(x=w1370, y=w1371) -> (x .or. y?=w1372:bool)
                  n204 = Or(x=w1360, y=w1361) -> (x .or. y?=w1353:bool)
                  n205 = Or(x=w1356, y=w1357) -> (x .or. y?=w1350:bool)
                  n206 = case shown="True" w1354 {
                    frame False {
                    }
                    frame True {
                      # "rechts"
                      # "links"
                      # "motor zwak rechts sneller"
                      n207 = xnode "Analog output (1 sample) 60"("B/AO1 (Pin 4)"=5.0) -> ()  [unwired: 1 in, 1 out]
                      n208 = xnode "Analog output (1 sample) 62"("A/AO0 (Pin 2)"=0.0) -> ()  [unwired: 1 in, 1 out]
                      n209 = xnode "Analog output (1 sample) 59"("B/AO0 (Pin 2)"=0.0) -> ()  [unwired: 1 in, 1 out]
                      n210 = xnode "Analog output (1 sample) 61"("A/AO1 (Pin 4)"=4.0) -> ()  [unwired: 1 in, 1 out]
                    }
                  }
                  n211 = case shown="True" w1352 {
                    frame False {
                    }
                    frame True {
                      # "rechts"
                      # "links"
                      # "motor zeer sterk rechts sneller"
                      n212 = xnode "Analog output (1 sample) 47"("B/AO1 (Pin 4)"=5.0) -> ()  [unwired: 1 in, 1 out]
                      n213 = xnode "Analog output (1 sample) 50"("A/AO0 (Pin 2)"=0.0) -> ()  [unwired: 1 in, 1 out]
                      n214 = xnode "Analog output (1 sample) 48"("B/AO0 (Pin 2)"=0.0) -> ()  [unwired: 1 in, 1 out]
                      n215 = xnode "Analog output (1 sample) 49"("A/AO1 (Pin 4)"=1.0) -> ()  [unwired: 1 in, 1 out]
                    }
                  }
                  n216 = case shown="True" w1375 {
                    frame False {
                    }
                    frame True {
                      # "rechts"
                      # "links"
                      # "motor  zeer sterk links sneller"
                      n217 = xnode "Analog output (1 sample) 70"("A/AO0 (Pin 2)"=0.0) -> ()  [unwired: 1 in, 1 out]
                      n218 = xnode "Analog output (1 sample) 68"("B/AO0 (Pin 2)"=0.0) -> ()  [unwired: 1 in, 1 out]
                      n219 = xnode "Analog output (1 sample) 67"("B/AO1 (Pin 4)"=1.0) -> ()  [unwired: 1 in, 1 out]
                      n220 = xnode "Analog output (1 sample) 69"("A/AO1 (Pin 4)"=5.0) -> ()  [unwired: 1 in, 1 out]
                    }
                  }
                  n221 = case shown="True" w1376 {
                    frame False {
                    }
                    frame True {
                      # "rechts"
                      # "links"
                      # "motor zwak links sneller"
                      n222 = xnode "Analog output (1 sample) 45"("A/AO1 (Pin 4)"=5.0) -> ()  [unwired: 1 in, 1 out]
                      n223 = xnode "Analog output (1 sample) 44"("B/AO0 (Pin 2)"=0.0) -> ()  [unwired: 1 in, 1 out]
                      n224 = xnode "Analog output (1 sample) 46"("A/AO0 (Pin 2)"=0.0) -> ()  [unwired: 1 in, 1 out]
                      n225 = xnode "Analog output (1 sample) 43"("B/AO1 (Pin 4)"=4.0) -> ()  [unwired: 1 in, 1 out]
                    }
                  }
                  n226 = case shown="True" w1364 {
                    frame False {
                    }
                    frame True {
                      # "rechts"
                      # "links"
                      # "motor naar links sneller"
                      n227 = xnode "Analog output (1 sample) 52"("B/AO0 (Pin 2)"=0.0) -> ()  [unwired: 1 in, 1 out]
                      n228 = xnode "Analog output (1 sample) 54"("A/AO0 (Pin 2)"=0.0) -> ()  [unwired: 1 in, 1 out]
                      n229 = xnode "Analog output (1 sample) 51"("B/AO1 (Pin 4)"=3.0) -> ()  [unwired: 1 in, 1 out]
                      n230 = xnode "Analog output (1 sample) 53"("A/AO1 (Pin 4)"=5.0) -> ()  [unwired: 1 in, 1 out]
                    }
                  }
                  n231 = case shown="True" w1372 {
                    frame False {
                    }
                    frame True {
                      # "rechts"
                      # "links"
                      # "motoren sterk links sneller"
                      n232 = xnode "Analog output (1 sample) 63"("B/AO1 (Pin 4)"=2.0) -> ()  [unwired: 1 in, 1 out]
                      n233 = xnode "Analog output (1 sample) 66"("A/AO0 (Pin 2)"=0.0) -> ()  [unwired: 1 in, 1 out]
                      n234 = xnode "Analog output (1 sample) 64"("B/AO0 (Pin 2)"=0.0) -> ()  [unwired: 1 in, 1 out]
                      n235 = xnode "Analog output (1 sample) 65"("A/AO1 (Pin 4)"=5.0) -> ()  [unwired: 1 in, 1 out]
                    }
                  }
                  n236 = case shown="True" w1353 {
                    frame False {
                    }
                    frame True {
                      # "rechts"
                      # "links"
                      # "motor naar rechts sneller"
                      n237 = xnode "Analog output (1 sample) 55"("B/AO1 (Pin 4)"=5.0) -> ()  [unwired: 1 in, 1 out]
                      n238 = xnode "Analog output (1 sample) 58"("A/AO0 (Pin 2)"=0.0) -> ()  [unwired: 1 in, 1 out]
                      n239 = xnode "Analog output (1 sample) 56"("B/AO0 (Pin 2)"=0.0) -> ()  [unwired: 1 in, 1 out]
                      n240 = xnode "Analog output (1 sample) 57"("A/AO1 (Pin 4)"=3.0) -> ()  [unwired: 1 in, 1 out]
                    }
                  }
                  n241 = case shown="True" w1350 {
                    frame False {
                    }
                    frame True {
                      # "rechts"
                      # "links"
                      # "motor sterk rechts sneller"
                      n242 = xnode "Analog output (1 sample) 27"("B/AO1 (Pin 4)"=5.0) -> ()  [unwired: 1 in, 1 out]
                      n243 = xnode "Analog output (1 sample) 28"("B/AO0 (Pin 2)"=0.0) -> ()  [unwired: 1 in, 1 out]
                      n244 = xnode "Analog output (1 sample) 30"("A/AO0 (Pin 2)"=0.0) -> ()  [unwired: 1 in, 1 out]
                      n245 = xnode "Analog output (1 sample) 29"("A/AO1 (Pin 4)"=2.0) -> ()  [unwired: 1 in, 1 out]
                    }
                  }
                }
                frame True {
                  n246 = xnode "Analog output (1 sample)"("A/AO0 (Pin 2)"=0) -> ()  [unwired: 1 in, 1 out]
                  n247 = xnode "Analog output (1 sample) 3"("B/AO0 (Pin 2)"=0) -> ()  [unwired: 1 in, 1 out]
                  n248 = xnode "Analog output (1 sample) 2"("A/AO1 (Pin 4)"=0) -> ()  [unwired: 1 in, 1 out]
                  n249 = xnode "Analog output (1 sample) 4"("B/AO1 (Pin 4)"=0) -> ()  [unwired: 1 in, 1 out]
                }
              }
            }
          }
        }
      }
    }
    n250 = feedback-in #1(w2) -> ()
  }
